vi "Drive Control Example - P vs PID.vi"() -> ()   [LabVIEW 2017]
uses:
  <vilib>/addons/control/pid/pid.llb/PID (DBL).vi
  <vilib>/addons/control/pid/NI_PID_pid.lvlib
panel:
  in  "D":dbl
  in  "I":dbl=10.0
  in  "P":dbl=0.3
  out "Motor Speed 2":dbl=1.0
  in  "stop 2":bool
  out "Dist From wall 2":dbl
  out "Waveform Chart 2":dbl(graph)
  in  "Sonar Distance 2":dbl=50.0
  in  "Enum":enum16{"P Control", "PID Control"}(ring)
  out "Waveform Chart":dbl(graph)
  out "Dist From wall":dbl
  in  "stop":bool
  in  "Sonar Distance":dbl=50.0
  out "Motor Speed":dbl=1.0
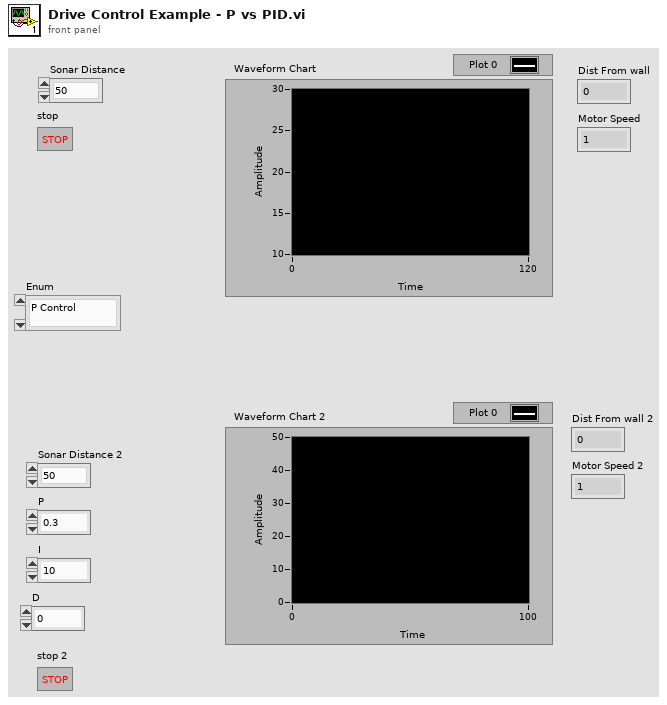
[diagram p1: front panel]
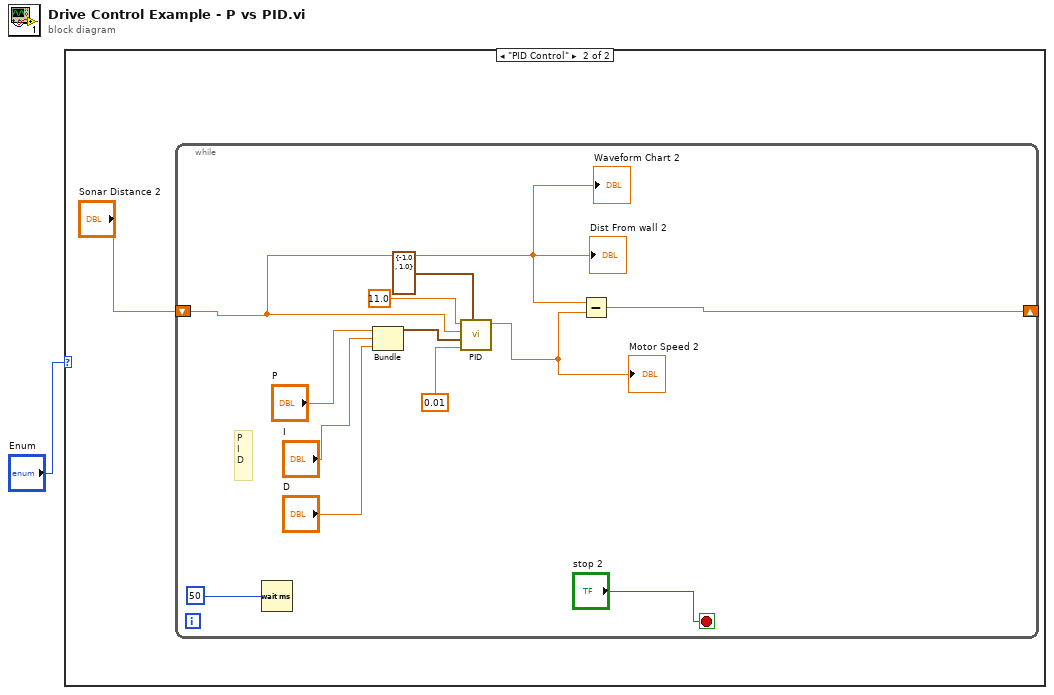
[diagram p0: block diagram]
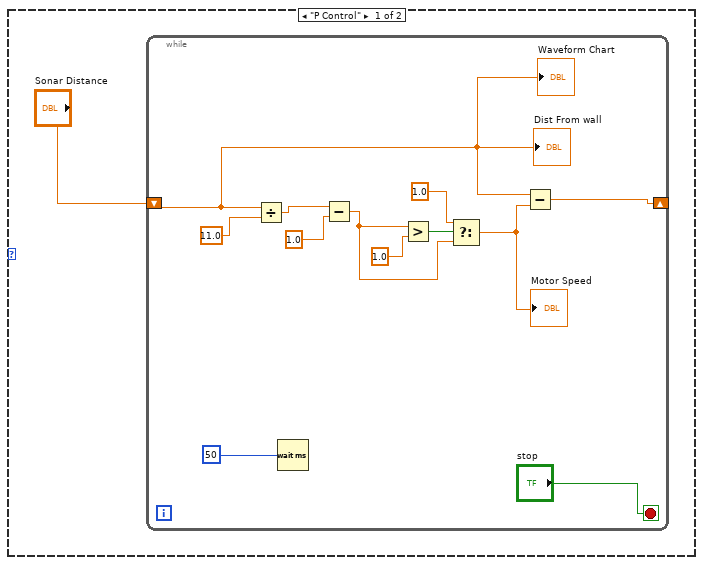
[diagram p2: hidden frame]
diagram:
  n1 = case shown="\"PID Control\"" "Enum" {
    frame "P Control" {
      n2 = while {
        shift-right: [w4] -> _
        shift-left: "Sonar Distance" -> [w3]
        stop <- "stop" stop-if-true
        n3 = Divide(x=w3, y=11.0) -> (x/y=w12:dbl)
        n4 = Wait (ms)(milliseconds to wait=50) -> ()  [unwired: 1 out]
        n5 = Subtract(x=w12, y=1.0) -> (x-y=w8:dbl)
        n6 = Greater?(x=w8, y=1.0) -> (0:w10:bool)
        n7 = Select(t=1.0, s=w10, f=w8) -> (s? t:f=w5:dbl)
        "Motor Speed" <- w5
        n8 = Subtract(x=w3, y=w5) -> (x-y=w4:dbl)
        "Dist From wall" <- w3
        "Waveform Chart" <- w3
      }
    }
    frame "PID Control" {
      n9 = while {
        shift-right: [w25] -> _
        shift-left: "Sonar Distance 2" -> [w18]
        stop <- "stop 2" stop-if-true
        # "P\nI\nD"
        n10 = Wait (ms)(milliseconds to wait=50) -> ()  [unwired: 1 out]
        n11 = Bundle("P"="P", "I"="I", "D"="D") -> (w24:cluster{"P":dbl, "I":dbl, "D":dbl})  [unwired: 1 in]
        n12 = call-poly <vilib>:"PID.vi"("output range"=cluster{"Lower value":sgl, "Upper value":sgl} {"Lower value"=-1.0, "Upper value"=1.0} ("Range"), "dt (s)"=0.01, "PID gains"=w24, "process variable"=w18, "setpoint"=11.0) -> ("output"=w17:dbl)  [unwired: 5 in, 1 out]
        "Motor Speed 2" <- w17
        n13 = Subtract(x=w18, y=w17) -> (x-y=w25:dbl)
        "Dist From wall 2" <- w18
        "Waveform Chart 2" <- w18
      }
    }
  }
